vi "Initialize.vi"(6 "optional":variant, 8 "error in":errorcluster, 11 "Parameters in":refnum<class "Parameters.lvclass">) -> (0 "error out":errorcluster, 3 "Node*":refnum<data-value>)   [LabVIEW 2013, in "Parameters.lvclass"]
doc: "Initializes a node. Makes a data value reference of the node, sets the selfNode, and output the data value reference."
uses:
  Parameters.lvclass
  xCE/xceNode/xceNode.lvclass
  xCE/xceDataNode/xceDataNode.lvclass
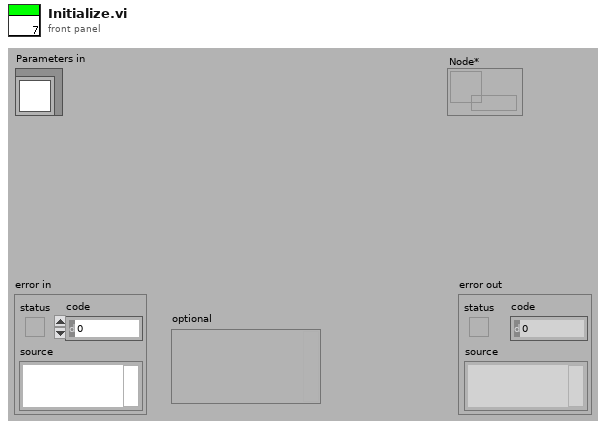
[diagram p1: front panel]
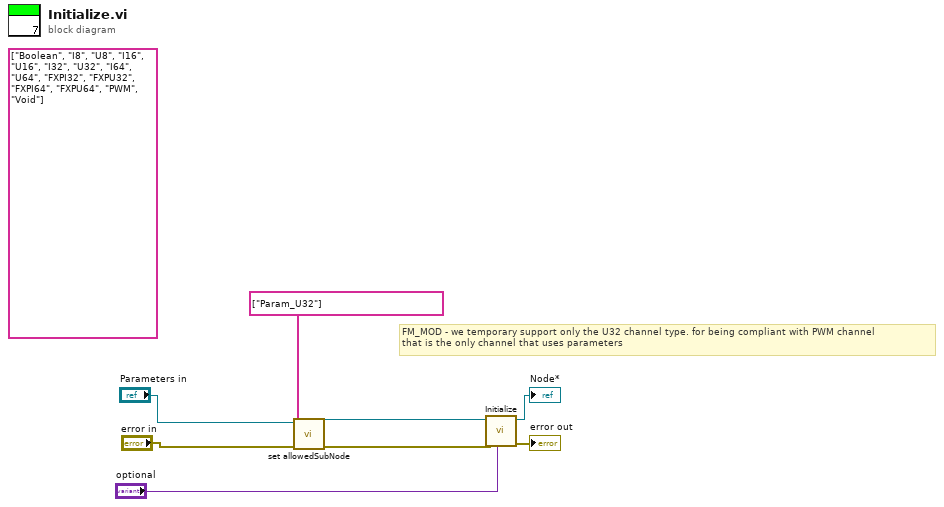
[diagram p0: block diagram]
diagram:
  (unwired) string[] ["Boolean", "I8", "U8", "I16", "U16", "I32", "U32", "I64", "U64", "FXPI32", "FXPU32", "FXPI64", "FXPU64", "PWM", "Void"] ("Allowed subNode[]")
  # "FM_MOD - we temporary support only the U32 channel type. for being compliant with PWM channel\nthat is the only channel that uses parameters"
  n1 = call "set allowedSubNode.vi"("error in (no error)"="error in", "Allowed subNode[]"=string[] ["Param_U32"], "xceDataNode in"="Parameters in") -> ("error out"=w3:errorcluster, "xceDataNode out"=w2:refnum<class "Parameters.lvclass">)  [unwired: 7 in]
  n2 = call-parent "Initialize.vi"("optional"="optional", "error in"=w3, "xceDataNode in"=w2) -> ("error out"=→"error out":errorcluster, "Node*"=→"Node*":refnum<data-value>)  [unwired: 7 in]
